vi "JSON text to Variant.vi"(4 "LVClass Serializer":refnum<class "JSONtext LVClass Serializer.lvclass">, 8 "error in (no error)":errorcluster, 9 "Data Type":variant, 10 "Offset":i32, 11 "JSON":string) -> (0 "error out":errorcluster, 1 "Variant out":variant)   [LabVIEW 2017, in "JSONtext.lvlib"]
doc: "Convert JSON to the Data Type entered, which may be a cluster or array."
uses:
  JSONtext.lvlib
  LVClass Serializer/JSONtext LVClass Serializer.lvclass
  <vilib>/Utility/Data Type/Type Definitions/Data Type.ctl
  support/Get String.vi
  support/Get Timestamp.vi
  support/Get I32.vi
  support/Get I64.vi
  support/Get U32.vi
  support/Get U64.vi
  support/Get Boolean.vi
  support/Get DBL.vi
  support/Get SGL.vi
  support/Unescape JSON string.vi
  support/quote and escape json string 2.vi
  Parsing/Advance past whitespace and comma.vi
  Parsing/Advance past next JSON Value (inlined COPY).vi
  Parsing/Advance past Item Name.vi
  Parsing/Advance past String.vi
  support/Get Number Text.vi
  Parsing/NaN or null to Integer ERROR.vi
  Parsing/Advance past Number.vi
  <vilib>/Utility/error.llb/Error Cluster From Error Code.vi
  <vilib>/Utility/Data Type/Get Refnum Information.vi
  support/Error Cluster From Code.vi
  <vilib>/JDP Science/JDP Science Common Utilities/Timestamp/Text to Timestamp.vi
  <vilib>/Utility/Data Type/Get Numeric Information.vi
  Parsing/Advance past Object.vi
  Parsing/Parsing Error.vi
  <vilib>/Utility/Data Type/NI_Data Type.lvlib
  <vilib>/JDP Science/JDP Science Common Utilities/JDP Utility.lvlib
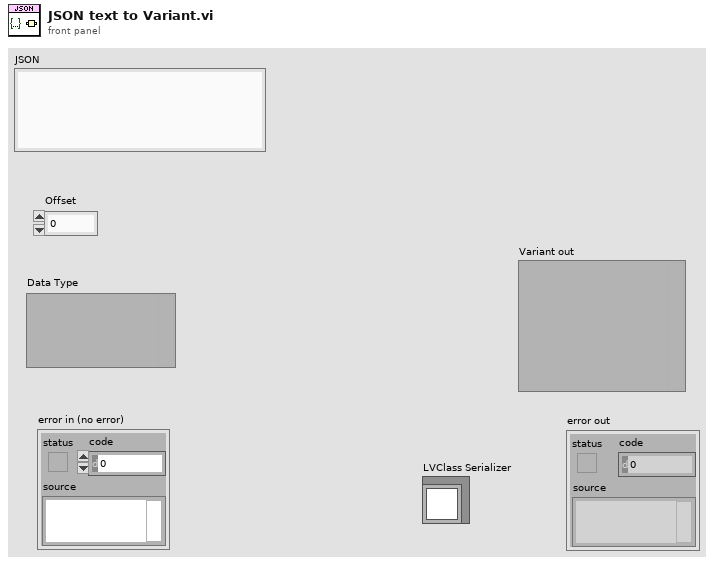
[diagram p1: front panel]
types:
  T1 = typedef "NI_Data Type.lvlib/Data Type.ctl" = enum8{"Invalid Type", "Void", "I8", "I16", "I32", "I64", "U8", "U16", "U32", "U64", "Single Float", "Double Float", "Extended Float", "Single Complex", "Double Complex", "Extended Complex", "Enum U8", "Enum U16", "Enum U32", "Enum U64", "Single Float With Unit", "Double Float With Unit", "Extended Float With Unit", "Single Complex with Unit", "Double Complex with Unit", "Extended Complex with Unit", "Boolean", "String", "Path", "Picture", "Tag", "Array", "Cluster", "Variant", "LV Variant", "Waveform", "Timestamp", "Digital Waveform", "Digital Data", "ExpressData", "Refnum", "External Data", "VI", "Poly VI", "LabVIEW Class Instance", "Fixed Point"}
  T2 = typedef "JSONtext.lvlib/Parsing State.ctl" = enum16{"Parser Error", "Object", "Array", "String", "Number/Other", "Leading Whitespace", "Object end", "Array end", "Value end"}
  T3 = typedef "JSONtext.lvlib/Tag Type.ctl" = enum16{"No Tag", "<JSON>", "<JOBJ>"}
  T4 = typedef "JSONtext.lvlib/JSON Value Type.ctl" = enum16{"Not a JSON Value", "JSON Object", "JSON Array", "String", "Number", "true", "false", "null"}
  T5 = typedef "JSONtext.lvlib/Found Items.ctl" = cluster{"Item offset":i32, "Offset past Item":i32, "Name offset":i32, "Offset past Name":i32, "Found":bool, "Item Type":T2, "Item Index":i32}
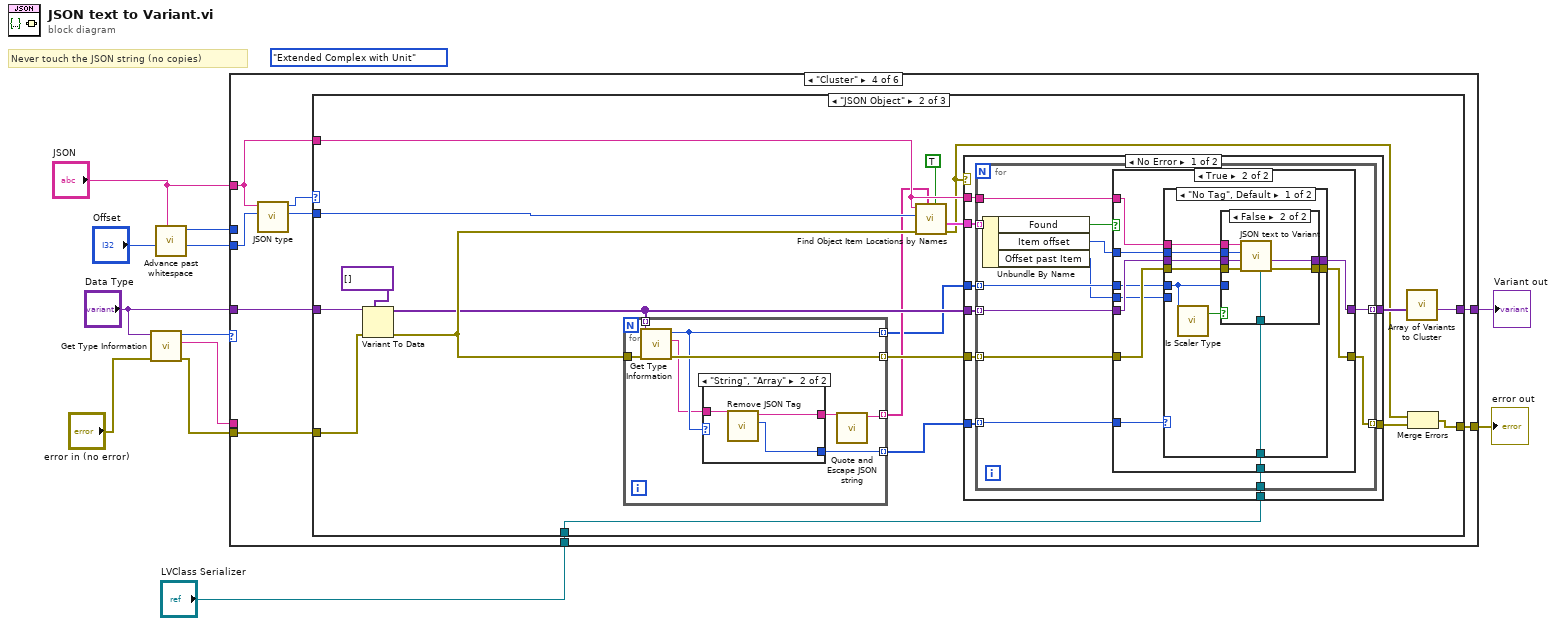
[diagram p0: block diagram]
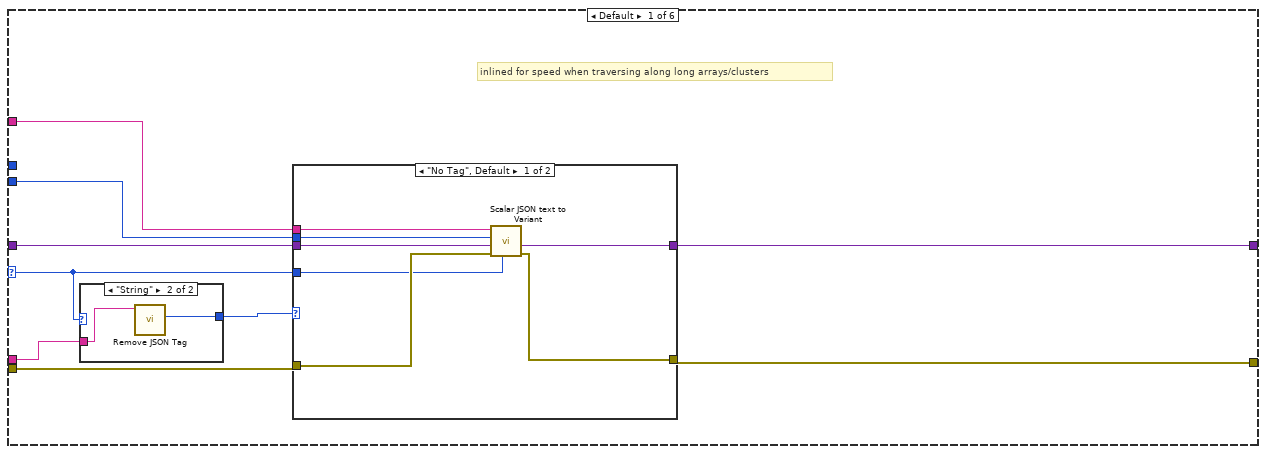
[diagram p2: hidden frame]
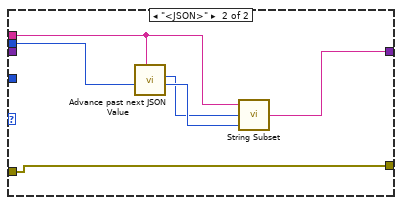
[diagram p3: hidden frame]
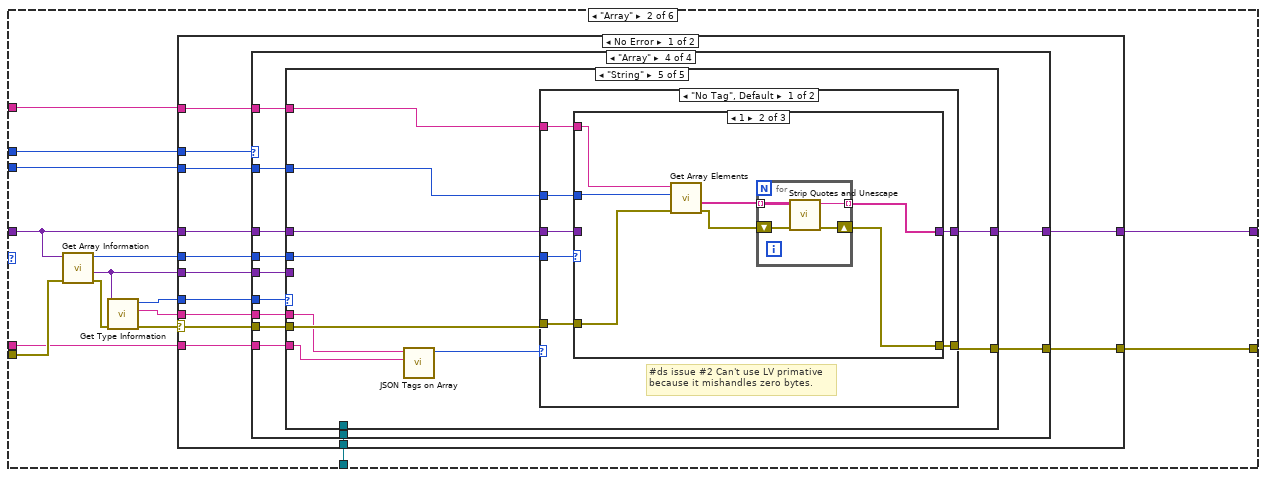
[diagram p5: hidden frame]
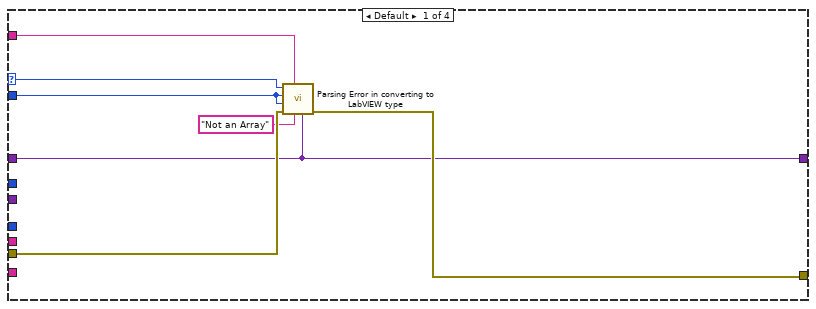
[diagram p6: hidden frame]
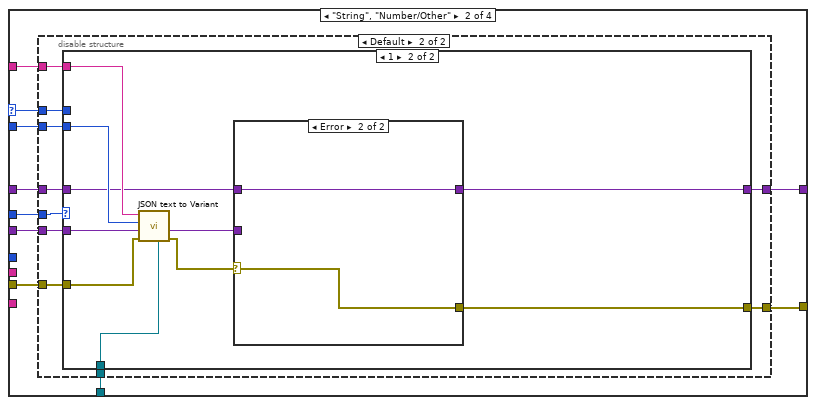
[diagram p7: hidden frame]
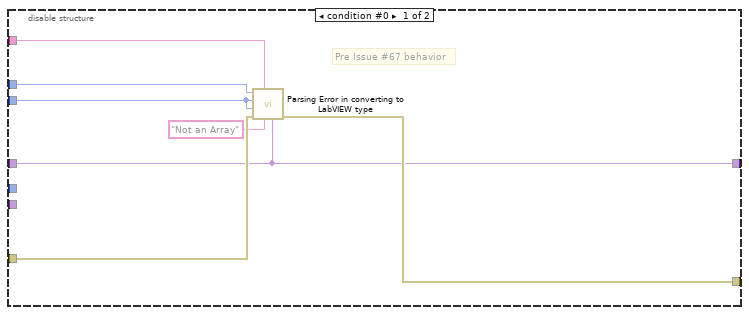
[diagram p8: hidden frame]
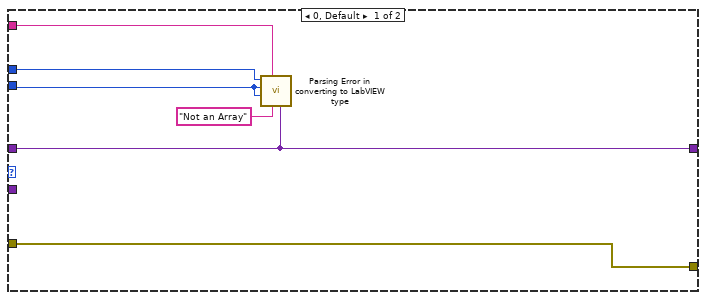
[diagram p9: hidden frame]
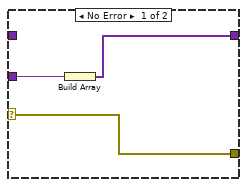
[diagram p10: hidden frame]
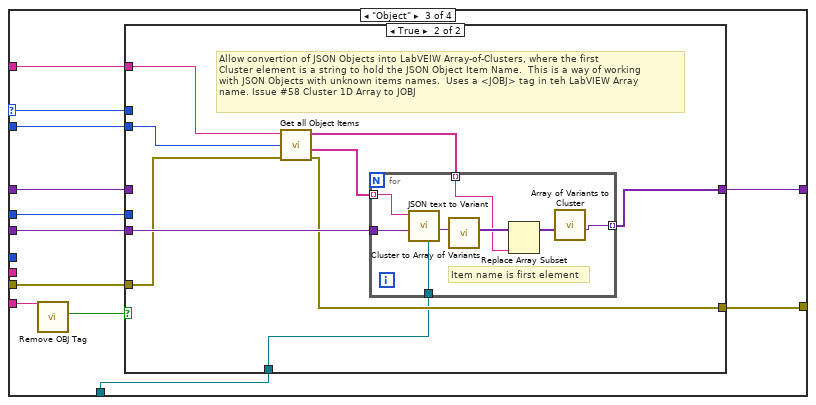
[diagram p11: hidden frame]
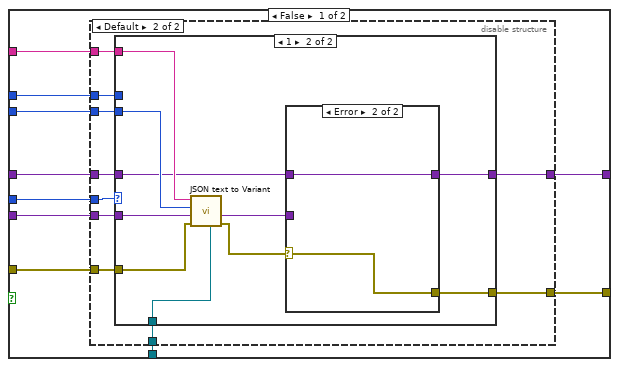
[diagram p12: hidden frame]
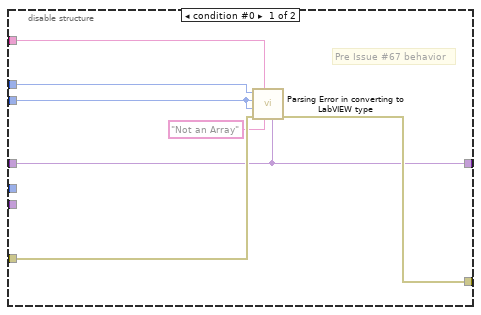
[diagram p13: hidden frame]
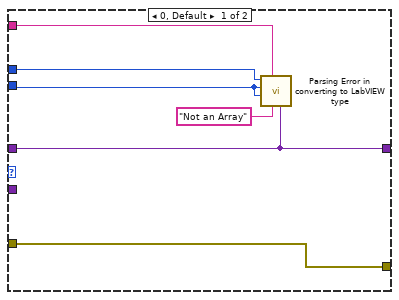
[diagram p14: hidden frame]
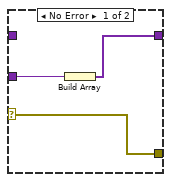
[diagram p15: hidden frame]
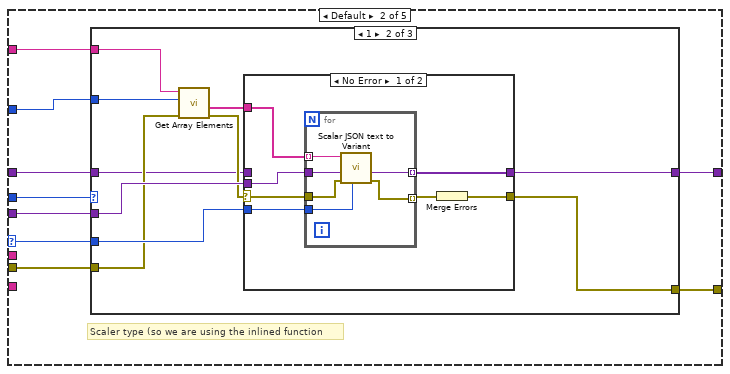
[diagram p17: hidden frame]
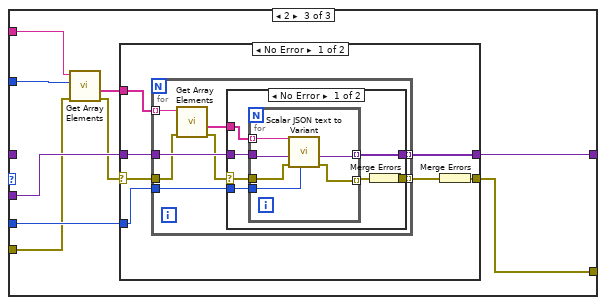
[diagram p20: hidden frame]
diagram:
  (unwired) Data_Type."Extended Complex with Unit" ("Type")
  # "Never touch the JSON string (no copies)"
  n1 = call <vilib>:"Get Type Information.vi"("error in (no error)"="error in (no error)", "Variant"="Data Type") -> ("error out"=w8:errorcluster, "Name"=w2:string, "Type"=w12:T1)  [unwired: 5 in, 2 out]
  n2 = call "Advance past whitespace.vi"("JSON"="JSON", "Offset"="Offset") -> ("Offset of first non-whitespace"=w5:i32, "Parser State"=w3:T2)  [unwired: 8 in]
  n3 = case shown="\"Cluster\"" w12 {
    selector: w12 -> [w14 _ _ _ _ _]
    tunnel: "Data Type" -> [w21 w44 w585 w594 w793 w801]
    tunnel: "JSON" -> [w19 w42 w578 w590 w788 w802]
    tunnel: [w16 w48 w575 w592 w785 w795] -> w9
    tunnel: w8 -> [w17 w51 w584 w593 w792 w799]
    tunnel: w5 -> [w18 w40 w577 w591 w787 w794]
    tunnel: [w20 w47 w568 w587 w790 w796] -> w7
    tunnel: w3 -> [_ w38 _ _ _ _]
    tunnel: w2 -> [w15 w41 _ _ _ _]
    tunnel: "LVClass Serializer" -> [_ w37 w567 w586 _ w803]
    frame Default {
      # "inlined for speed when traversing along long arrays/clusters"
      n4 = case shown="\"String\"" w14 {
        tunnel: w15 -> [_ w36]
        tunnel: [_ w35] -> w13
        frame "Invalid Type", Default {
        }
        frame "String" {
          n5 = call "Remove JSON Tag.vi"("Name"=w36) -> ("Tag"=w35:T3)  [unwired: 9 in, 1 out]
        }
      }
      n6 = case shown="\"No Tag\", Default" w13 {
        tunnel: w21 -> [w28 _]
        tunnel: [w27 w30] -> w20
        tunnel: w19 -> [w26 w31]
        tunnel: w18 -> [w25 w34]
        tunnel: w17 -> [w24 w29]
        tunnel: [w23 w29] -> w16
        tunnel: w14 -> [w22 _]
        frame "No Tag", Default {
          n7 = call "Scalar JSON text to Variant.vi"("Type"=w22, "error in (no error)"=w24, "Variant (Data Type)"=w28, "Offset"=w25, "JSON"=w26) -> ("error out"=w23:errorcluster, "Variant out"=w27:variant)  [unwired: 5 in]
        }
        frame "<JSON>" {
          n8 = call "Advance past next JSON Value.vi"("JSON"=w31, "Offset"=w34) -> ("Offset out"=w33:i32, "Value start"=w32:i32)  [unwired: 7 in, 1 out]
          n9 = call "String Subset.vi"("Offset past End"=w33, "Start offset"=w32, "JSON"=w31) -> ("substring"=w30:string)  [unwired: 2 in]
        }
      }
    }
    frame "Array" {
      n10 = call <vilib>:"Get Array Information.vi"("error in (no error)"=w51, "Variant"=w44) -> ("error out"=w50:errorcluster, "Array Element Data Type"=w43:variant, "Number of Dimensions"=w45:i32)  [unwired: 6 in, 1 out]
      n11 = call <vilib>:"Get Type Information.vi"("error in (no error)"=w50, "Variant"=w43) -> ("error out"=w49:errorcluster, "Name"=w39:string, "Type"=w46:T1)  [unwired: 5 in, 2 out]
      n12 = case shown="No Error" w49 {
        selector: w49 -> [w64 w566]
        tunnel: [w63 w566] -> w48
        tunnel: [w62 w565] -> w47
        tunnel: w46 -> [w61 _]
        tunnel: w45 -> [w60 _]
        tunnel: w44 -> [w59 w565]
        tunnel: w43 -> [w58 _]
        tunnel: w42 -> [w57 _]
        tunnel: w41 -> [w56 _]
        tunnel: w40 -> [w55 _]
        tunnel: w39 -> [w54 _]
        tunnel: w38 -> [w53 _]
        tunnel: w37 -> [w52 _]
        frame No Error {
          n13 = case shown="\"Array\"" w53 {
            selector: w53 -> [w69 w79 w129 _]
            tunnel: w64 -> [w68 w78 w128 w208]
            tunnel: [w67 w77 w127 w207] -> w63
            tunnel: [w66 w74 w124 w206] -> w62
            tunnel: w61 -> [_ _ _ w205]
            tunnel: w60 -> [_ w73 w123 w204]
            tunnel: w59 -> [w66 w76 w126 w203]
            tunnel: w58 -> [_ w75 w125 w202]
            tunnel: w57 -> [w71 w81 w131 w201]
            tunnel: w56 -> [_ _ w121 w200]
            tunnel: w55 -> [w70 w80 w130 w199]
            tunnel: w54 -> [_ _ _ w198]
            tunnel: w52 -> [_ w72 w122 w197]
            frame Default {
              n14 = call "Parsing Error in converting to LabVIEW type.vi"("LV Type"=w66, "initial string"="Not an Array", "JSON"=w71, "error in (no error)"=w68, "Offset past match"=w70, "Value start"=w70, "State"=w69) -> ("error out"=w67:errorcluster)  [unwired: 4 in]
            }
            frame "String", "Number/Other" {
              n15 = disable-structure shown="Default" {
                disable-tunnel: w81 -> [w88 w97]
                disable-tunnel: w80 -> [w87 w96]
                disable-tunnel: w79 -> [w86 w90]
                disable-tunnel: w78 -> [w85 w95]
                disable-tunnel: [w84 w92] -> w77
                disable-tunnel: w76 -> [w82 w93]
                disable-tunnel: w75 -> [_ w98]
                disable-tunnel: [w82 w94] -> w74
                disable-tunnel: w73 -> [_ w91]
                disable-tunnel: w72 -> [_ w89]
                frame condition #0 {
                  # "Pre Issue #67 behavior"
                  n16 = call "Parsing Error in converting to LabVIEW type.vi"("LV Type"=w82, "initial string"="Not an Array", "JSON"=w88, "error in (no error)"=w85, "Offset past match"=w87, "Value start"=w87, "State"=w86) -> ("error out"=w84:errorcluster)  [unwired: 4 in]
                }
                frame condition #1 (active) {
                  n17 = case shown="1" w91 {
                    tunnel: w98 -> [_ w114]
                    tunnel: w97 -> [w103 w113]
                    tunnel: w96 -> [w101 w112]
                    tunnel: w95 -> [w99 w110]
                    tunnel: [w100 w108] -> w94
                    tunnel: w93 -> [w100 w107]
                    tunnel: [w99 w106] -> w92
                    tunnel: w90 -> [w102 _]
                    tunnel: w89 -> [_ w105]
                    frame 0, Default {
                      n18 = call "Parsing Error in converting to LabVIEW type.vi"("LV Type"=w100, "initial string"="Not an Array", "JSON"=w103, "Offset past match"=w101, "Value start"=w101, "State"=w102) -> ()  [unwired: 5 in, 1 out]
                    }
                    frame 1 {
                      n19 = call "JSON text to Variant.vi"("LVClass Serializer"=w105, "error in (no error)"=w110, "Data Type"=w114, "Offset"=w112, "JSON"=w113) -> ("error out"=w109:errorcluster, "Variant out"=w111:variant)  [unwired: 5 in]
                      n20 = case shown="Error" w109 {
                        selector: w109 -> [w115 w118]
                        tunnel: w111 -> [w117 _]
                        tunnel: [w116 w119] -> w108
                        tunnel: w107 -> [_ w119]
                        tunnel: [w115 w118] -> w106
                        frame No Error {
                          n21 = Build Array(w117) -> (w116:variant[])
                        }
                        frame Error {
                        }
                      }
                    }
                  }
                }
              }
            }
            frame "Object" {
              n22 = call "Remove OBJ Tag.vi"("Name"=w121) -> ("tagged as Item Name in JSON Objects"=w120:bool)  [unwired: 9 in, 1 out]
              n23 = case shown="True" w120 {
                tunnel: w131 -> [w141 w186]
                tunnel: w130 -> [w140 w180]
                tunnel: w129 -> [w139 _]
                tunnel: w128 -> [w138 w187]
                tunnel: [w137 w184] -> w127
                tunnel: w126 -> [w136 _]
                tunnel: w125 -> [w135 w188]
                tunnel: [w134 w185] -> w124
                tunnel: w123 -> [w133 _]
                tunnel: w122 -> [w132 w183]
                frame False {
                  n24 = disable-structure shown="Default" {
                    disable-tunnel: w141 -> [w148 w157]
                    disable-tunnel: w140 -> [w147 w156]
                    disable-tunnel: w139 -> [w146 w150]
                    disable-tunnel: w138 -> [w145 w155]
                    disable-tunnel: [w144 w152] -> w137
                    disable-tunnel: w136 -> [w142 w153]
                    disable-tunnel: w135 -> [_ w158]
                    disable-tunnel: [w142 w154] -> w134
                    disable-tunnel: w133 -> [_ w151]
                    disable-tunnel: w132 -> [_ w149]
                    frame condition #0 {
                      # "Pre Issue #67 behavior"
                      n25 = call "Parsing Error in converting to LabVIEW type.vi"("LV Type"=w142, "initial string"="Not an Array", "JSON"=w148, "error in (no error)"=w145, "Offset past match"=w147, "Value start"=w147, "State"=w146) -> ("error out"=w144:errorcluster)  [unwired: 4 in]
                    }
                    frame condition #1 (active) {
                      n26 = case shown="1" w151 {
                        tunnel: w158 -> [_ w174]
                        tunnel: w157 -> [w163 w173]
                        tunnel: w156 -> [w161 w172]
                        tunnel: w155 -> [w159 w170]
                        tunnel: [w160 w168] -> w154
                        tunnel: w153 -> [w160 w167]
                        tunnel: [w159 w166] -> w152
                        tunnel: w150 -> [w162 _]
                        tunnel: w149 -> [_ w165]
                        frame 0, Default {
                          n27 = call "Parsing Error in converting to LabVIEW type.vi"("LV Type"=w160, "initial string"="Not an Array", "JSON"=w163, "Offset past match"=w161, "Value start"=w161, "State"=w162) -> ()  [unwired: 5 in, 1 out]
                        }
                        frame 1 {
                          n28 = call "JSON text to Variant.vi"("LVClass Serializer"=w165, "error in (no error)"=w170, "Data Type"=w174, "Offset"=w172, "JSON"=w173) -> ("error out"=w169:errorcluster, "Variant out"=w171:variant)  [unwired: 5 in]
                          n29 = case shown="Error" w169 {
                            selector: w169 -> [w175 w178]
                            tunnel: w171 -> [w177 _]
                            tunnel: [w176 w179] -> w168
                            tunnel: w167 -> [_ w179]
                            tunnel: [w175 w178] -> w166
                            frame No Error {
                              n30 = Build Array(w177) -> (w176:variant[])
                            }
                            frame Error {
                            }
                          }
                        }
                      }
                    }
                  }
                }
                frame True {
                  # "Allow convertion of JSON Objects into LabVEIW Array-of-Clusters, where the first\nCluster element is a string to hold the JSON Object Item Name.  This is a way of working\nwith JSON Objects with unknown items names.  Uses a <JOBJ> tag in teh LabVIEW Array\nname. Issue #58 Cluster 1D Array to JOBJ"
                  n31 = call "Get all Object Items.vi"("error in (no error)"=w187, "Offset"=w180, "JSON"=w186) -> ("error out"=w184:errorcluster, "<JSON>"=w182:string[], "Item Names"=w181:string[])  [unwired: 5 in, 1 out]
                  n32 = for {
                    tunnel: w182 -> [w196] mode=indexing
                    tunnel: w188 -> [w195]
                    tunnel: w181 -> [w191] mode=indexing
                    tunnel: [w190] -> w185 mode=indexing
                    tunnel: w183 -> [w189]
                    # "Item name is first element"
                    n33 = call "JSON text to Variant.vi"("LVClass Serializer"=w189, "Data Type"=w195, "JSON"=w196) -> ("Variant out"=w193:variant)  [unwired: 7 in, 1 out]
                    n34 = call <vilib>:"Cluster to Array of Variants.vi"("Cluster"=w193) -> ("Array of Cluster Elements"=w192:variant[])  [unwired: 10 in]
                    n35 = Replace Array Subset(array=w192, new element=w191) -> (w194:variant[])  [unwired: 1 in]
                    n36 = call <vilib>:"Array of Variants to Cluster.vi"("Array of Variants"=w194) -> ("Cluster of Variants"=w190:variant)  [unwired: 10 in]
                  }
                }
              }
            }
            frame "Array" {
              n37 = case shown="\"String\"" w205 {
                selector: w205 -> [_ w211 _ w374 _]
                tunnel: w201 -> [_ w215 w293 w372 w502]
                tunnel: w208 -> [w209 w218 w296 w379 w501]
                tunnel: [w209 w219 w297 w378 w500] -> w207
                tunnel: [w210 w216 w294 w377 w499] -> w206
                tunnel: w204 -> [_ w214 w292 w376 w498]
                tunnel: w203 -> [w210 w213 w291 w375 w497]
                tunnel: w202 -> [_ w217 w295 _ _]
                tunnel: w199 -> [_ w212 w290 w371 w495]
                tunnel: w200 -> [_ _ w289 _ w496]
                tunnel: w198 -> [_ _ _ _ w494]
                tunnel: w197 -> [_ _ w288 _ _]
                frame "Invalid Type" {
                }
                frame Default {
                  # "Scaler type (so we are using the inlined function"
                  n38 = case shown="1" w214 {
                    tunnel: [w220 w231 w250] -> w219
                    tunnel: w218 -> [w220 w224 w248]
                    tunnel: w217 -> [_ w230 w255]
                    tunnel: [w221 w228 w253] -> w216
                    tunnel: w212 -> [_ w227 w252]
                    tunnel: w215 -> [_ w226 w251]
                    tunnel: w213 -> [w221 w222 _]
                    tunnel: w211 -> [_ w225 w249]
                    frame 0, Default {
                    }
                    frame 1 {
                      n39 = call "Get Array Elements.vi"("error in (no error)"=w224, "Offset"=w227, "JSON"=w226) -> ("error out"=w223:errorcluster, "<JSON>"=w229:string[])  [unwired: 6 in, 1 out]
                      n40 = case shown="No Error" w223 {
                        selector: w223 -> [w232 w245]
                        tunnel: [w237 w245] -> w231
                        tunnel: w230 -> [w236 _]
                        tunnel: w229 -> [w235 _]
                        tunnel: [w234 w246] -> w228
                        tunnel: w225 -> [w233 _]
                        tunnel: w222 -> [_ w246]
                        frame No Error {
                          n41 = for {
                            tunnel: w236 -> [w243]
                            tunnel: w232 -> [w241]
                            tunnel: [w240] -> w238 mode=indexing
                            tunnel: [w242] -> w234 mode=indexing
                            tunnel: w235 -> [w244] mode=indexing
                            tunnel: w233 -> [w239]
                            n42 = call "Scalar JSON text to Variant.vi"("Type"=w239, "error in (no error)"=w241, "Variant (Data Type)"=w243, "JSON"=w244) -> ("error out"=w240:errorcluster, "Variant out"=w242:variant)  [unwired: 6 in]
                          }
                          n43 = Merge Errors(w238) -> (w237:errorcluster)
                        }
                        frame Error {
                        }
                      }
                    }
                    frame 2 {
                      n44 = call "Get Array Elements.vi"("error in (no error)"=w248, "Offset"=w252, "JSON"=w251) -> ("error out"=w247:errorcluster, "<JSON>"=w254:string[])  [unwired: 6 in, 1 out]
                      n45 = case shown="No Error" w247 {
                        selector: w247 -> [w256 w287]
                        tunnel: w255 -> [w261 w286]
                        tunnel: w254 -> [w260 _]
                        tunnel: [w259 w286] -> w253
                        tunnel: [w258 w287] -> w250
                        tunnel: w249 -> [w257 _]
                        frame No Error {
                          n46 = for {
                            tunnel: [w270] -> w262 mode=indexing
                            tunnel: w256 -> [w264]
                            tunnel: w261 -> [w269]
                            tunnel: w260 -> [w267] mode=indexing
                            tunnel: [w268] -> w259 mode=indexing
                            tunnel: w257 -> [w265]
                            n47 = call "Get Array Elements.vi"("error in (no error)"=w264, "JSON"=w267) -> ("error out"=w263:errorcluster, "<JSON>"=w266:string[])  [unwired: 7 in, 1 out]
                            n48 = case shown="No Error" w263 {
                              selector: w263 -> [w271 w284]
                              tunnel: [w276 w284] -> w270
                              tunnel: w269 -> [w275 w285]
                              tunnel: [w274 w285] -> w268
                              tunnel: w266 -> [w273 _]
                              tunnel: w265 -> [w272 _]
                              frame No Error {
                                n49 = for {
                                tunnel: w275 -> [w279]
                                tunnel: w271 -> [w280]
                                tunnel: [w281] -> w277 mode=indexing
                                tunnel: [w282] -> w274 mode=indexing
                                tunnel: w273 -> [w283] mode=indexing
                                tunnel: w272 -> [w278]
                                n50 = call "Scalar JSON text to Variant.vi"("Type"=w278, "error in (no error)"=w280, "Variant (Data Type)"=w279, "JSON"=w283) -> ("error out"=w281:errorcluster, "Variant out"=w282:variant)  [unwired: 6 in]
                                }
                                n51 = Merge Errors(w277) -> (w276:errorcluster)
                              }
                              frame Error {
                              }
                            }
                          }
                          n52 = Merge Errors(w262) -> (w258:errorcluster)
                        }
                        frame Error {
                        }
                      }
                    }
                  }
                }
                frame "Cluster".."Waveform", "LabVIEW Class Instance" {
                  n53 = case shown="1" w292 {
                    tunnel: [w298 w309 w329] -> w297
                    tunnel: w296 -> [w298 w308 w328]
                    tunnel: w295 -> [_ w307 w334]
                    tunnel: [w299 w306 w332] -> w294
                    tunnel: w290 -> [_ w304 w331]
                    tunnel: w293 -> [_ w305 w330]
                    tunnel: w291 -> [w299 w303 w326]
                    tunnel: w289 -> [_ _ _]
                    tunnel: w288 -> [_ w302 w325]
                    frame 0, Default {
                    }
                    frame 1 {
                      n54 = call "Get Array Elements.vi"("error in (no error)"=w308, "Offset"=w304, "JSON"=w305) -> ("error out"=w300:errorcluster, "<JSON>"=w301:string[])  [unwired: 6 in, 1 out]
                      n55 = case shown="No Error" w300 {
                        selector: w300 -> [w311 w324]
                        tunnel: [w315 w324] -> w309
                        tunnel: w307 -> [w314 _]
                        tunnel: [w313 w323] -> w306
                        tunnel: w301 -> [w312 _]
                        tunnel: w303 -> [_ w323]
                        tunnel: w302 -> [w310 _]
                        frame No Error {
                          n56 = for {
                            tunnel: w314 -> [w322]
                            tunnel: w311 -> [w321]
                            tunnel: [w320] -> w316 mode=indexing
                            tunnel: [w319] -> w313 mode=indexing
                            tunnel: w312 -> [w318] mode=indexing
                            tunnel: w310 -> [w317]
                            n57 = call "JSON text to Variant.vi"("LVClass Serializer"=w317, "error in (no error)"=w321, "Data Type"=w322, "JSON"=w318) -> ("error out"=w320:errorcluster, "Variant out"=w319:variant)  [unwired: 6 in]
                          }
                          n58 = Merge Errors(w316) -> (w315:errorcluster)
                        }
                        frame Error {
                        }
                      }
                    }
                    frame 2 {
                      n59 = call "Get Array Elements.vi"("error in (no error)"=w328, "Offset"=w331, "JSON"=w330) -> ("error out"=w327:errorcluster, "<JSON>"=w333:string[])  [unwired: 6 in, 1 out]
                      n60 = case shown="No Error" w327 {
                        selector: w327 -> [w337 w368]
                        tunnel: w334 -> [w341 _]
                        tunnel: w333 -> [w340 _]
                        tunnel: [w339 w367] -> w332
                        tunnel: [w338 w368] -> w329
                        tunnel: w326 -> [w336 w367]
                        tunnel: w325 -> [w335 _]
                        frame No Error {
                          n61 = for {
                            tunnel: [w351] -> w342 mode=indexing
                            tunnel: w337 -> [w346]
                            tunnel: w341 -> [w350]
                            tunnel: w340 -> [w348] mode=indexing
                            tunnel: [w349] -> w339 mode=indexing
                            tunnel: w336 -> [w344]
                            tunnel: w335 -> [w343]
                            n62 = call "Get Array Elements.vi"("error in (no error)"=w346, "JSON"=w348) -> ("error out"=w345:errorcluster, "<JSON>"=w347:string[])  [unwired: 7 in, 1 out]
                            n63 = case shown="No Error" w345 {
                              selector: w345 -> [w353 w366]
                              tunnel: [w357 w366] -> w351
                              tunnel: w350 -> [w356 _]
                              tunnel: [w355 w365] -> w349
                              tunnel: w347 -> [w354 _]
                              tunnel: w344 -> [_ w365]
                              tunnel: w343 -> [w352 _]
                              frame No Error {
                                n64 = for {
                                tunnel: w356 -> [w364]
                                tunnel: w353 -> [w363]
                                tunnel: [w362] -> w358 mode=indexing
                                tunnel: [w361] -> w355 mode=indexing
                                tunnel: w354 -> [w360] mode=indexing
                                tunnel: w352 -> [w359]
                                n65 = call "JSON text to Variant.vi"("LVClass Serializer"=w359, "error in (no error)"=w363, "Data Type"=w364, "JSON"=w360) -> ("error out"=w362:errorcluster, "Variant out"=w361:variant)  [unwired: 6 in]
                                }
                                n66 = Merge Errors(w358) -> (w357:errorcluster)
                              }
                              frame Error {
                              }
                            }
                          }
                          n67 = Merge Errors(w342) -> (w338:errorcluster)
                        }
                        frame Error {
                        }
                      }
                    }
                  }
                }
                frame "I8".."Extended Complex", "Single Float With Unit".."Extended Float With Unit" {
                  # "Use LV JSON primative for speed"
                  n68 = call "Advance past Array.vi"("JSON"=w372, "Offset"=w371) -> ("Offset past Array"=w373:i32, "Empty Array"=w369:bool, "Array Start"=w370:i32)  [unwired: 6 in, 1 out]
                  n69 = case shown="False" w369 {
                    tunnel: w379 -> [w389 w492]
                    tunnel: [w388 w492] -> w378
                    tunnel: [w387 w491] -> w377
                    tunnel: w376 -> [w386 _]
                    tunnel: w375 -> [w385 w491]
                    tunnel: w374 -> [w383 _]
                    tunnel: w373 -> [w382 _]
                    tunnel: w372 -> [w381 _]
                    tunnel: w370 -> [w380 _]
                    frame False {
                      n70 = call "String Subset.vi"("Offset past End"=w382, "Start offset"=w380, "JSON"=w381) -> ("substring"=w384:string)  [unwired: 2 in]
                      n71 = case shown="3" w386 {
                        tunnel: w384 -> [_ w397 w430 w463]
                        tunnel: w389 -> [w390 w396 w429 w462]
                        tunnel: [w390 w395 w428 w461] -> w388
                        tunnel: [w391 w393 w426 w459] -> w387
                        tunnel: w385 -> [w391 w392 w425 w458]
                        tunnel: w383 -> [_ w394 w427 w460]
                        frame 0, Default {
                        }
                        frame 1 {
                          n72 = case shown="\"I8\"..\"I32\"" w394 {
                            tunnel: w397 -> [_ w404 w409 w414 w419 w424]
                            tunnel: w396 -> [w398 w402 w407 w412 w417 w422]
                            tunnel: [w398 w401 w406 w411 w416 w421] -> w395
                            tunnel: [w399 w400 w405 w410 w415 w420] -> w393
                            tunnel: w392 -> [w399 _ _ _ _ _]
                            frame "Invalid Type", Default {
                            }
                            frame "Single Float".."Extended Float", "Single Float With Unit".."Extended Float With Unit" {
                              n73 = Unflatten From JSON(JSON string=w404, type and defaults=dbl[] [], error in (no error)=w402) -> (value=w400:dbl[], error out=w401:errorcluster)  [unwired: 4 in]
                            }
                            frame "U8".."U32" {
                              n74 = Unflatten From JSON(JSON string=w409, type and defaults=u32[] [], error in (no error)=w407) -> (value=w405:u32[], error out=w406:errorcluster)  [unwired: 4 in]
                            }
                            frame "U64" {
                              n75 = Unflatten From JSON(JSON string=w414, type and defaults=u64[] [], error in (no error)=w412) -> (value=w410:u64[], error out=w411:errorcluster)  [unwired: 4 in]
                            }
                            frame "I8".."I32" {
                              n76 = Unflatten From JSON(JSON string=w419, type and defaults=i32[] [], error in (no error)=w417) -> (value=w415:i32[], error out=w416:errorcluster)  [unwired: 4 in]
                            }
                            frame "I64" {
                              n77 = Unflatten From JSON(JSON string=w424, type and defaults=i64[] [], error in (no error)=w422) -> (value=w420:i64[], error out=w421:errorcluster)  [unwired: 4 in]
                            }
                          }
                        }
                        frame 2 {
                          n78 = case shown="\"Single Float\"..\"Extended Float\", \"Single Float With Unit\"..\"Extended Float With Unit\"" w427 {
                            tunnel: w430 -> [_ w437 w442 w447 w452 w457]
                            tunnel: w429 -> [w431 w435 w440 w445 w450 w455]
                            tunnel: [w431 w434 w439 w444 w449 w454] -> w428
                            tunnel: [w432 w433 w438 w443 w448 w453] -> w426
                            tunnel: w425 -> [w432 _ _ _ _ _]
                            frame "Invalid Type", Default {
                            }
                            frame "Single Float".."Extended Float", "Single Float With Unit".."Extended Float With Unit" {
                              n79 = Unflatten From JSON(JSON string=w437, type and defaults=dbl[][] [], error in (no error)=w435) -> (value=w433:dbl[][], error out=w434:errorcluster)  [unwired: 4 in]
                            }
                            frame "U8".."U32" {
                              n80 = Unflatten From JSON(JSON string=w442, type and defaults=u32[][] [], error in (no error)=w440) -> (value=w438:u32[][], error out=w439:errorcluster)  [unwired: 4 in]
                            }
                            frame "U64" {
                              n81 = Unflatten From JSON(JSON string=w447, type and defaults=u64[][] [], error in (no error)=w445) -> (value=w443:u64[][], error out=w444:errorcluster)  [unwired: 4 in]
                            }
                            frame "I8".."I32" {
                              n82 = Unflatten From JSON(JSON string=w452, type and defaults=i32[][] [], error in (no error)=w450) -> (value=w448:i32[][], error out=w449:errorcluster)  [unwired: 4 in]
                            }
                            frame "I64" {
                              n83 = Unflatten From JSON(JSON string=w457, type and defaults=i64[][] [], error in (no error)=w455) -> (value=w453:i64[][], error out=w454:errorcluster)  [unwired: 4 in]
                            }
                          }
                        }
                        frame 3 {
                          n84 = case shown="\"I8\"..\"I32\"" w460 {
                            tunnel: w463 -> [_ w470 w475 w480 w485 w490]
                            tunnel: w462 -> [w464 w468 w473 w478 w483 w488]
                            tunnel: [w464 w467 w472 w477 w482 w487] -> w461
                            tunnel: [w465 w466 w471 w476 w481 w486] -> w459
                            tunnel: w458 -> [w465 _ _ _ _ _]
                            frame "Invalid Type", Default {
                            }
                            frame "Single Float".."Extended Float", "Single Float With Unit".."Extended Float With Unit" {
                              n85 = Unflatten From JSON(JSON string=w470, type and defaults=dbl[][][] [], error in (no error)=w468) -> (value=w466:dbl[][][], error out=w467:errorcluster)  [unwired: 4 in]
                            }
                            frame "U8".."U32" {
                              n86 = Unflatten From JSON(JSON string=w475, type and defaults=u32[][][] [], error in (no error)=w473) -> (value=w471:u32[][][], error out=w472:errorcluster)  [unwired: 4 in]
                            }
                            frame "U64" {
                              n87 = Unflatten From JSON(JSON string=w480, type and defaults=u64[][][] [], error in (no error)=w478) -> (value=w476:u64[][][], error out=w477:errorcluster)  [unwired: 4 in]
                            }
                            frame "I8".."I32" {
                              n88 = Unflatten From JSON(JSON string=w485, type and defaults=i32[][][] [], error in (no error)=w483) -> (value=w481:i32[][][], error out=w482:errorcluster)  [unwired: 4 in]
                            }
                            frame "I64" {
                              n89 = Unflatten From JSON(JSON string=w490, type and defaults=i64[][][] [], error in (no error)=w488) -> (value=w486:i64[][][], error out=w487:errorcluster)  [unwired: 4 in]
                            }
                          }
                        }
                      }
                    }
                    frame True {
                    }
                  }
                }
                frame "String" {
                  n90 = call "JSON Tags on Array.vi"("Array Name"=w496, "Element Name"=w494) -> ("Tag"=w493:T3)  [unwired: 9 in]
                  n91 = case shown="\"No Tag\", Default" w493 {
                    tunnel: w502 -> [w509 w546]
                    tunnel: w501 -> [w508 w545]
                    tunnel: [w507 w544] -> w500
                    tunnel: [w506 w543] -> w499
                    tunnel: w498 -> [w505 w542]
                    tunnel: w497 -> [w504 w541]
                    tunnel: w495 -> [w503 w540]
                    frame "No Tag", Default {
                      # "#ds issue #2 Can't use LV primative\nbecause it mishandles zero bytes."
                      n92 = case shown="1" w505 {
                        tunnel: w509 -> [_ w516 w524]
                        tunnel: w508 -> [w510 w513 w525]
                        tunnel: [w510 w514 w526] -> w507
                        tunnel: [w511 w515 w527] -> w506
                        tunnel: w504 -> [w511 _ _]
                        tunnel: w503 -> [_ w512 w523]
                        frame 0, Default {
                        }
                        frame 1 {
                          n93 = call "Get Array Elements.vi"("error in (no error)"=w513, "Offset"=w512, "JSON"=w516) -> ("error out"=w518:errorcluster, "<JSON>"=w517:string[])  [unwired: 6 in, 1 out]
                          n94 = for {
                            tunnel: w517 -> [w522] mode=indexing
                            tunnel: [w521] -> w515 mode=indexing
                            shift-right: [w520] -> w514
                            shift-left: w518 -> [w519]
                            n95 = call "Strip Quotes and Unescape.vi"("error in (no error)"=w519, "String"=w522) -> ("error out"=w520:errorcluster, "result string"=w521:string)  [unwired: 8 in]
                          }
                        }
                        frame 2 {
                          n96 = call "Get Array Elements.vi"("error in (no error)"=w525, "Offset"=w523, "JSON"=w524) -> ("error out"=w529:errorcluster, "<JSON>"=w528:string[])  [unwired: 6 in, 1 out]
                          n97 = for {
                            tunnel: w528 -> [w535] mode=indexing
                            tunnel: [w532] -> w527 mode=indexing
                            shift-right: [w531] -> w526
                            shift-left: w529 -> [w534]
                            n98 = call "Get Array Elements.vi"("error in (no error)"=w534, "JSON"=w535) -> ("error out"=w530:errorcluster, "<JSON>"=w533:string[])  [unwired: 7 in, 1 out]
                            n99 = for {
                              tunnel: w533 -> [w539] mode=indexing
                              tunnel: [w538] -> w532 mode=indexing
                              shift-right: [w537] -> w531
                              shift-left: w530 -> [w536]
                              n100 = call "Strip Quotes and Unescape.vi"("error in (no error)"=w536, "String"=w539) -> ("error out"=w537:errorcluster, "result string"=w538:string)  [unwired: 8 in]
                            }
                          }
                        }
                      }
                    }
                    frame "<JSON>" {
                      # "JSON text"
                      n101 = case shown="2" w542 {
                        tunnel: w546 -> [_ w553 w555]
                        tunnel: w545 -> [w547 w552 w556]
                        tunnel: [w547 w551 w557] -> w544
                        tunnel: [w548 w550 w558] -> w543
                        tunnel: w541 -> [w548 _ _]
                        tunnel: w540 -> [_ w549 w554]
                        frame 0, Default {
                        }
                        frame 1 {
                          n102 = call "Get Array Elements.vi"("error in (no error)"=w552, "Offset"=w549, "JSON"=w553) -> ("error out"=w551:errorcluster, "<JSON>"=w550:string[])  [unwired: 6 in, 1 out]
                        }
                        frame 2 {
                          n103 = call "Get Array Elements.vi"("error in (no error)"=w556, "Offset"=w554, "JSON"=w555) -> ("error out"=w560:errorcluster, "<JSON>"=w559:string[])  [unwired: 6 in, 1 out]
                          n104 = for {
                            tunnel: w559 -> [w564] mode=indexing
                            tunnel: [w561] -> w558 mode=indexing
                            shift-right: [w562] -> w557
                            shift-left: w560 -> [w563]
                            n105 = call "Get Array Elements.vi"("error in (no error)"=w563, "JSON"=w564) -> ("error out"=w562:errorcluster, "<JSON>"=w561:string[])  [unwired: 7 in, 1 out]
                          }
                        }
                      }
                    }
                  }
                }
              }
            }
          }
        }
        frame Error {
        }
      }
    }
    frame "Waveform" {
      # "Attributes not supported"
      n106 = Variant To Data(error in=w584, type=waveform(dbl) {"t0"=timestamp(0 s since 1904-01-01), "dt"=1.0, "Y"=[]} ("waveform"), Variant=w585) -> (data=w582:waveform(dbl), error out=w576:errorcluster)
      n107 = Unbundle By Name(w582) -> ("t0"=w581:timestamp, "dt"=w580:dbl, "Y"=w579:dbl[])  [unwired: 1 out]
      n108 = Bundle("t0"=w581, "dt"=w580, "Y"=w579) -> (w573:cluster{"t0":timestamp, "dt":dbl, "Y":dbl[]})  [unwired: 1 in]
      n109 = call "JSON text to Variant.vi"("LVClass Serializer"=w567, "error in (no error)"=w576, "Data Type"=w573, "Offset"=w577, "JSON"=w578) -> ("error out"=w575:errorcluster, "Variant out"=w574:variant)  [unwired: 5 in]
      n110 = Variant To Data(type=w573, Variant=w574) -> (data=w572:cluster{"t0":timestamp, "dt":dbl, "Y":dbl[]})  [unwired: 1 in, 1 out]
      n111 = Unbundle By Name(w572) -> ("t0"=w571:timestamp, "dt"=w570:dbl, "Y"=w569:dbl[])
      n112 = Bundle By Name("t0"=w571, "dt"=w570, "Y"=w569) -> (w568:waveform(dbl))  [unwired: 1 in]
    }
    frame "Cluster" {
      n113 = call "JSON type.vi"("Offset"=w591, "JSON"=w590) -> ("Item Offset"=w589:i32, "JSON Value Type"=w588:T4)  [unwired: 8 in]
      n114 = case shown="\"JSON Object\"" w588 {
        selector: w588 -> [w599 _ w713]
        tunnel: w594 -> [w596 w620 w723]
        tunnel: w593 -> [w595 w618 w721]
        tunnel: [w596 w607 w714] -> w587
        tunnel: [w597 w616 w720] -> w592
        tunnel: w590 -> [_ w613 w717]
        tunnel: w589 -> [_ w612 w716]
        tunnel: w586 -> [_ w602 w712]
        frame Default {
          # "Issue #65"
          n115 = Format Into String(w599) -> (resulting string=w598:string)  [unwired: 3 in, 1 out]
          n116 = call "Format Error.vi"("error code (402842)"=402844, "error in (no error)"=w595, "message part 2"=w598, "error message"="Cannot Get as a Cluster: " ("format string")) -> ("error out"=w597:errorcluster)  [unwired: 7 in]
        }
        frame "JSON Object" {
          n117 = Variant To Data(error in=w618, type=variant[] [], Variant=w620) -> (data=w614:variant[], error out=w615:errorcluster)
          n118 = for {
            tunnel: w614 -> [w707] mode=indexing
            tunnel: w615 -> [w706]
            tunnel: [w705] -> w611 mode=indexing
            tunnel: [w703] -> w608 mode=indexing
            tunnel: [w704] -> w610 mode=indexing
            tunnel: [w701] -> w609 mode=indexing
            n119 = call <vilib>:"Get Type Information.vi"("error in (no error)"=w706, "Variant"=w707) -> ("error out"=w705:errorcluster, "Name"=w702:string, "Type"=w703:T1)  [unwired: 5 in, 2 out]
            n120 = case shown="\"String\", \"Array\"" w703 {
              tunnel: w702 -> [w708 w711]
              tunnel: [_ w710] -> w704
              tunnel: [w708 w709] -> w700
              frame Default {
              }
              frame "String", "Array" {
                n121 = call "Remove JSON Tag.vi"("Name"=w711) -> ("Tag"=w710:T3, "Name (tag stripped)"=w709:string)  [unwired: 9 in]
              }
            }
            n122 = call "Quote and Escape JSON string.vi"("Plain Text"=w700) -> ("<JSON>"=w701:string)  [unwired: 10 in]
          }
          n123 = call "Find Object Item Locations by Names.vi"("Insertion point if not found"=TRUE, "Item Names <JSON>"=w609, "error in (no error)"=w615, "Object Offset"=w612, "JSON"=w613) -> ("error out"=w603:errorcluster, "Items"=w605:T5[])  [unwired: 5 in]
          n124 = case shown="No Error" w603 {
            tunnel: [w629 w698] -> w606
            tunnel: [w628 w699] -> w617
            tunnel: w611 -> [w627 w698]
            tunnel: w605 -> [w626 _]
            tunnel: w610 -> [w625 _]
            tunnel: w608 -> [w624 _]
            tunnel: w614 -> [w623 w699]
            tunnel: w613 -> [w622 _]
            tunnel: w602 -> [w621 _]
            frame No Error {
              n125 = for {
                tunnel: w623 -> [w641] mode=indexing
                tunnel: w622 -> [w640]
                tunnel: [w639] -> w629 mode=indexing
                tunnel: [w638] -> w628 mode=indexing
                tunnel: w627 -> [w637] mode=indexing
                tunnel: w624 -> [w636] mode=indexing
                tunnel: w626 -> [w635] mode=indexing
                tunnel: w625 -> [w631] mode=indexing
                tunnel: w621 -> [w630]
                n126 = Unbundle By Name(w635) -> ("Found"=w634:bool, "Item offset"=w633:i32, "Offset past Item"=w632:i32)
                n127 = case shown="True" w634 {
                  tunnel: w640 -> [_ w653]
                  tunnel: w633 -> [_ w652]
                  tunnel: w641 -> [w643 w651]
                  tunnel: [w643 w647] -> w638
                  tunnel: w637 -> [w642 w650]
                  tunnel: [w642 w649] -> w639
                  tunnel: w636 -> [_ w648]
                  tunnel: w632 -> [_ w645]
                  tunnel: w631 -> [_ w646]
                  tunnel: w630 -> [_ w644]
                  frame False {
                  }
                  frame True {
                    n128 = case shown="\"No Tag\", Default" w646 {
                      tunnel: w653 -> [w662 w685]
                      tunnel: w652 -> [w661 w684]
                      tunnel: w651 -> [w660 w678]
                      tunnel: w650 -> [w659 w680]
                      tunnel: [w658 w679] -> w649
                      tunnel: w648 -> [w655 w681]
                      tunnel: [w657 w682] -> w647
                      tunnel: w645 -> [_ w683]
                      tunnel: w644 -> [w654 w677]
                      frame "No Tag", Default {
                        n129 = call "Is Scaler Type.vi"("Type"=w655) -> ("Scaler Type"=w656:bool)  [unwired: 2 in]
                        n130 = case shown="False" w656 {
                          tunnel: w662 -> [w669 w676]
                          tunnel: w661 -> [w668 w675]
                          tunnel: [w667 w674] -> w657
                          tunnel: w660 -> [w665 w673]
                          tunnel: w659 -> [w664 w672]
                          tunnel: [w666 w671] -> w658
                          tunnel: w655 -> [w663 _]
                          tunnel: w654 -> [_ w670]
                          frame True {
                            n131 = call "Scalar JSON text to Variant.vi"("Type"=w663, "error in (no error)"=w664, "Variant (Data Type)"=w665, "Offset"=w668, "JSON"=w669) -> ("error out"=w666:errorcluster, "Variant out"=w667:variant)  [unwired: 5 in]
                          }
                          frame False {
                            n132 = call "JSON text to Variant.vi"("LVClass Serializer"=w670, "error in (no error)"=w672, "Data Type"=w673, "Offset"=w675, "JSON"=w676) -> ("error out"=w671:errorcluster, "Variant out"=w674:variant)  [unwired: 5 in]
                          }
                        }
                      }
                      frame "<JSON>" {
                        # "<JSON>"
                        n133 = case shown="\"Array\"" w681 {
                          tunnel: w685 -> [w692 w697]
                          tunnel: w684 -> [w691 w696]
                          tunnel: w683 -> [_ w695]
                          tunnel: [w688 w694] -> w682
                          tunnel: w680 -> [w689 w693]
                          tunnel: [w687 w693] -> w679
                          tunnel: w678 -> [w690 _]
                          tunnel: w677 -> [w686 _]
                          frame "Array" {
                            n134 = call "JSON text to Variant.vi"("LVClass Serializer"=w686, "error in (no error)"=w689, "Data Type"=w690, "Offset"=w691, "JSON"=w692) -> ("error out"=w687:errorcluster, "Variant out"=w688:variant)  [unwired: 5 in]
                          }
                          frame "String", Default {
                            n135 = call "String Subset.vi"("Offset past End"=w695, "Start offset"=w696, "JSON"=w697) -> ("substring"=w694:string)  [unwired: 2 in]
                          }
                        }
                      }
                    }
                  }
                }
              }
            }
            frame Error {
              # "Issue 40"
            }
          }
          n136 = call <vilib>:"Array of Variants to Cluster.vi"("Array of Variants"=w617) -> ("Cluster of Variants"=w607:variant)  [unwired: 10 in]
          n137 = Merge Errors(w603, w606) -> (w616:errorcluster)
        }
        frame "JSON Array" {
          n138 = Variant To Data(error in=w721, type=variant[] [], Variant=w723) -> (data=w718:variant[], error out=w719:errorcluster)
          n139 = call "Possible Ragged Array.vi"("Array"=w718) -> ("Ragged Array posible"=w715:bool)  [unwired: 10 in]
          n140 = case shown="False" w715 {
            tunnel: [w737 w777] -> w720
            tunnel: w716 -> [w725 w780]
            tunnel: w719 -> [w736 w778]
            tunnel: w718 -> [w729 w783]
            tunnel: w717 -> [w728 w781]
            tunnel: [w726 w775] -> w714
            tunnel: w713 -> [w735 _]
            tunnel: w712 -> [w724 w774]
            frame False {
              # "First Cluster Element Unnamed"
              n141 = Index Array(array=w729) -> (element=w734:variant)  [unwired: 1 in]
              n142 = call <vilib>:"Get Type Information.vi"("Variant"=w734) -> ("Name"=w731:string, "Type"=w732:T1)  [unwired: 6 in, 3 out]
              n143 = case shown="\"String\", \"Array\"" w732 {
                tunnel: w731 -> [w738 w740]
                tunnel: [w738 w739] -> w733
                frame Default {
                }
                frame "String", "Array" {
                  n144 = call "Remove JSON Tag.vi"("Name"=w740) -> ("Name (tag stripped)"=w739:string)  [unwired: 9 in, 1 out]
                }
              }
              n145 = Empty String/Path?(string/path=w733) -> (empty?=w730:bool)
              n146 = case shown="True" w730 {
                tunnel: [w744 w755] -> w737
                tunnel: w736 -> [w743 w750]
                tunnel: w735 -> [w742 _]
                tunnel: [w741 w752] -> w727
                tunnel: w729 -> [w741 w754]
                tunnel: w728 -> [_ w753]
                tunnel: w725 -> [_ w751]
                tunnel: w724 -> [_ w748]
                frame False {
                  n147 = Format Into String(w742) -> (resulting string=w745:string)  [unwired: 3 in, 1 out]
                  n148 = call "Format Error.vi"("error code (402842)"=402844, "error in (no error)"=w743, "message part 2"=w745, "error message"="Cannot Get Array as a Cluster: " ("format string")) -> ("error out"=w744:errorcluster)  [unwired: 7 in]
                }
                frame True {
                  # "Unnamed cluster elements\n--> JSON Array"
                  n149 = call "Get Array Elements.vi"("error in (no error)"=w750, "Offset"=w751, "JSON"=w753) -> ("error out"=w749:errorcluster, "<JSON>"=w756:string[])  [unwired: 6 in, 1 out]
                  n150 = for {
                    tunnel: w754 -> [w765] mode=indexing
                    tunnel: w749 -> [w763]
                    tunnel: [w762] -> w757 mode=indexing
                    tunnel: [w764] -> w752 mode=indexing
                    tunnel: w756 -> [w761]
                    tunnel: w748 -> [w758]
                    i -> [w759]
                    n151 = Index Array(array=w761, index=w759) -> (element=w760:string)
                    n152 = case shown="Default" w760 {
                      selector: w760 -> [_ w769]
                      tunnel: w765 -> [w767 w773]
                      tunnel: [w767 w772] -> w764
                      tunnel: w763 -> [w766 w771]
                      tunnel: [w766 w770] -> w762
                      tunnel: w758 -> [_ w768]
                      frame "" {
                      }
                      frame Default {
                        n153 = call "JSON text to Variant.vi"("LVClass Serializer"=w768, "error in (no error)"=w771, "Data Type"=w773, "JSON"=w769) -> ("error out"=w770:errorcluster, "Variant out"=w772:variant)  [unwired: 6 in]
                      }
                    }
                  }
                  n154 = Merge Errors(w757) -> (w755:errorcluster)
                }
              }
              n155 = call <vilib>:"Array of Variants to Cluster.vi"("Array of Variants"=w727) -> ("Cluster of Variants"=w726:variant)  [unwired: 10 in]
            }
            frame True {
              # "Let a JSON Array be valid for an Array as sole element in a Cluster, as this is a way of doing \"Ragged\" arrays in LabVIEW."
              n156 = Index Array(array=w783) -> (element=w782:variant)  [unwired: 1 in]
              n157 = call "JSON text to Variant.vi"("LVClass Serializer"=w774, "error in (no error)"=w778, "Data Type"=w782, "Offset"=w780, "JSON"=w781) -> ("error out"=w777:errorcluster, "Variant out"=w779:variant)  [unwired: 5 in]
              n158 = Build Array(w779) -> (w776:variant[])
              n159 = call <vilib>:"Array of Variants to Cluster.vi"("Array of Variants"=w776) -> ("Cluster of Variants"=w775:variant)  [unwired: 10 in]
            }
          }
        }
      }
    }
    frame "Variant", "LV Variant" {
      # "Unwrap and rewrap"
      n160 = Variant To Data(error in=w792, type=variant, Variant=w793) -> (data=w784:variant, error out=w789:errorcluster)
      n161 = call "JSON text to Variant.vi"("error in (no error)"=w789, "Data Type"=w784, "Offset"=w787, "JSON"=w788) -> ("error out"=w785:errorcluster, "Variant out"=w786:variant)  [unwired: 6 in]
      n162 = To Variant(anything=w786) -> (Variant=w790:variant)
    }
    frame "LabVIEW Class Instance" {
      # "Issue #56 Way of providing alternate format\nof LVObjects"
      n163 = Variant To Data(error in=w799, type=refnum<class> refnum ("LabVIEW Object"), Variant=w801) -> (data=w797:refnum<class>, error out=w800:errorcluster)
      n164 = call-dynamic "JSON to LVObject.vi"("JSONtext LVClass Serializer in"=w803, "error in (no error)"=w800, "Object Type"=w797, "Offset"=w794, "JSON"=w802) -> ("error out"=w795:errorcluster, "Object"=w796:refnum<class>)  [unwired: 5 in]
    }
  }
  "Variant out" <- w7
  "error out" <- w9
